vi "back_propagation.vi"(5 "Y":dbl[](array[numeric]), 7 "X":dbl[][](array[numeric]), 8 "W2":dbl[][](array[numeric]), 9 "Z1":dbl[][](array[numeric]), 10 "A2":dbl[][](array[numeric]), 11 "A1":dbl[][](array[numeric])) -> (0 "db2":dbl[](array[numeric]), 1 "dW2":dbl[][](array[numeric]), 2 "db1":dbl[](array[numeric]), 3 "dW1":dbl[][](array[numeric]))   [LabVIEW 2023]
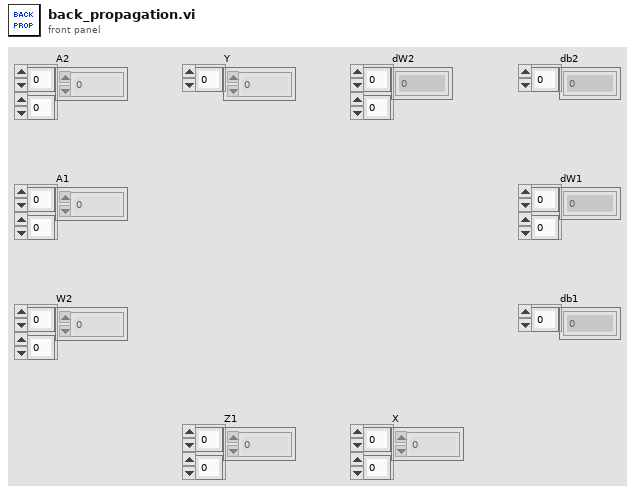
[diagram p1: front panel]
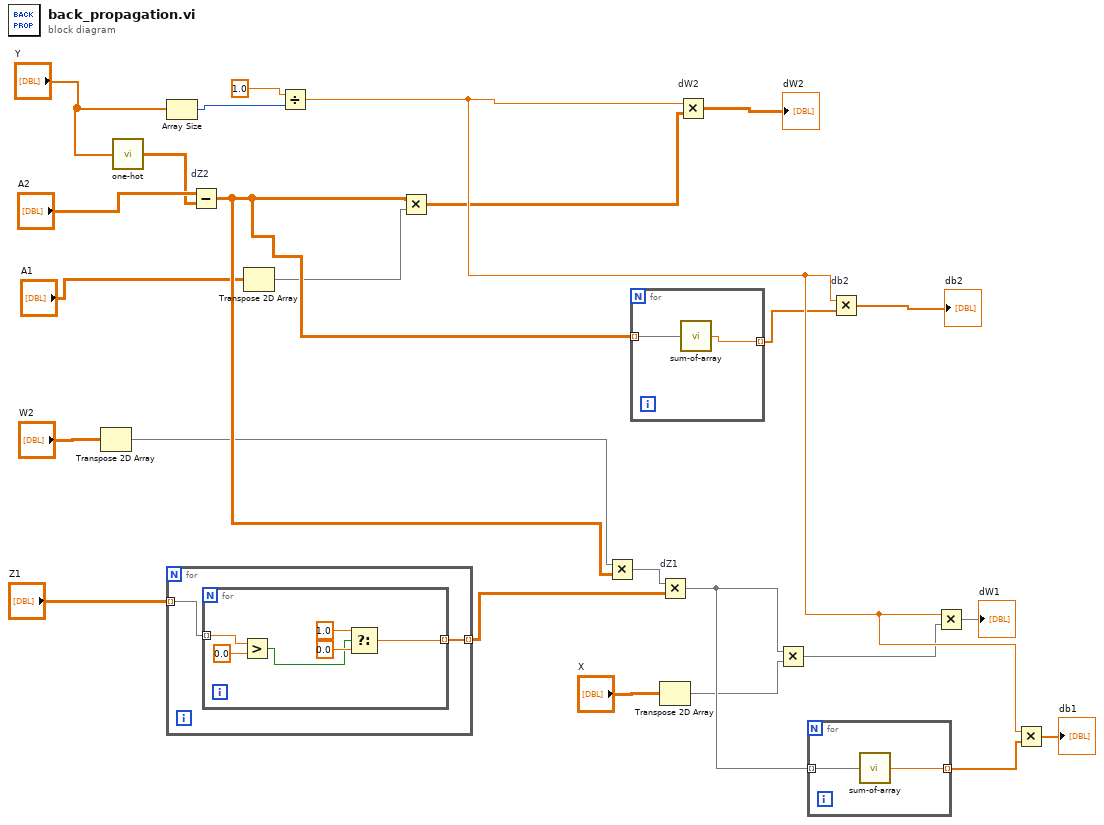
[diagram p0: block diagram]
diagram:
  n1 = Transpose 2D Array(2D array="W2") -> (transposed array=w14:dbl[][])
  n2 = call "one-hot.vi"("array"="Y") -> ("transposed array"=w2:dbl[][])
  n3 = Array Size(array="Y") -> (size(s)=w6:i32)
  n4 = for {
    tunnel: [w27] -> w17 mode=indexing
    tunnel: "Z1" -> [w26] mode=indexing
    n5 = for {
      tunnel: w26 -> [w29] mode=indexing
      tunnel: [w28] -> w27 mode=indexing
      n6 = Greater?(x=w29, y=0.0) -> (0:w31:bool)
      n7 = Select(t=1.0, s=w31, f=0.0) -> (s? t:f=w28:dbl)
    }
  }
  n8 = Subtract "dZ2"(x="A2", y=w2) -> (x-y=w15:dbl[][])
  n9 = Transpose 2D Array(2D array="A1") -> (transposed array=w10:dbl[][])
  n10 = Divide(x=1.0, y=w6) -> (x/y=w23:dbl)
  n11 = Multiply(x=w15, y=w10) -> (x*y=w11:dbl[][])
  n12 = Multiply ("ddd")(x=w14, y=w15) -> (x*y=w16:dbl[][])
  n13 = for {
    tunnel: w15 -> [w35] mode=indexing
    tunnel: [w34] -> w7 mode=indexing
    n14 = call "sum-of-array.vi"("Array"=w35) -> ("sum of array"=w34:dbl)
  }
  n15 = Multiply "dZ1"(x=w16, y=w17) -> (x*y=w22:dbl[][])
  n16 = Transpose 2D Array(2D array="X") -> (transposed array=w19:dbl[][])
  n17 = Multiply "dW2"(x=w23, y=w11) -> (x*y=→"dW2":dbl[][])
  n18 = Multiply ("ddd")(x=w22, y=w19) -> (x*y=w20:dbl[][])
  n19 = for {
    tunnel: w22 -> [w37] mode=indexing
    tunnel: [w36] -> w24 mode=indexing
    n20 = call "sum-of-array.vi"("Array"=w37) -> ("sum of array"=w36:dbl)
  }
  n21 = Multiply "db2"(x=w23, y=w7) -> (x*y=→"db2":dbl[])
  n22 = Multiply(x=w23, y=w20) -> (x*y=→"dW1":dbl[][])
  n23 = Multiply(x=w23, y=w24) -> (x*y=→"db1":dbl[])
